vi "test variant to json cluster.vi"(8 "error in (no error)":errorcluster) -> (0 "error out":errorcluster)   [LabVIEW 2019, in "labview_json_tests.lvlib"]
uses:
  labview_json_tests.lvlib
  lib/labview_json.lvlib
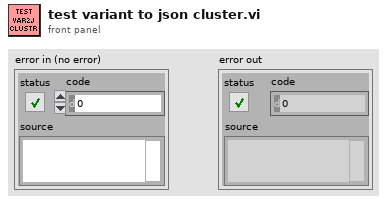
[diagram p1: front panel]
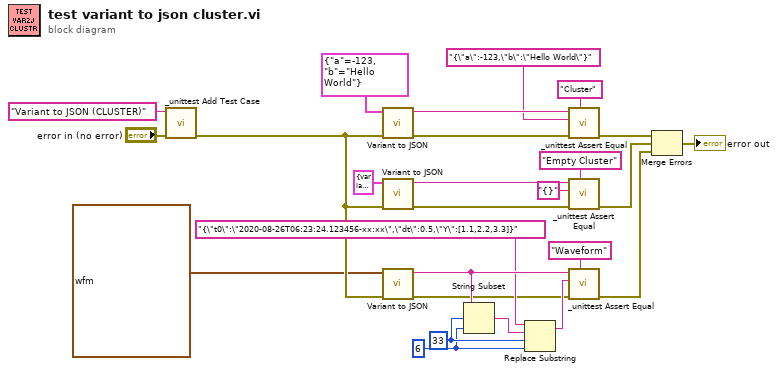
[diagram p0: block diagram]
diagram:
  w5 = 6 ("length (len. of substring)")
  w6 = 33 ("offset (0)")
  n1 = call "_unittest Add Test Case.vi"("error in (no error)"="error in (no error)", "Test Case"="Variant to JSON (CLUSTER)") -> ("error out"=w9:errorcluster)  [unwired: 9 in]
  n2 = call "Variant to JSON.vi"("error in (no error)"=w9, "Variant in"=cluster{"a":i32, "b":string} {"a"=-123, "b"="Hello World"} ("Cluster")) -> ("error out"=w21:errorcluster, "JSON"=w20:string)  [unwired: 8 in]
  n3 = call "Variant to JSON.vi"("error in (no error)"=w9, "Variant in"=cluster{variant} {variant} ("Cluster")) -> ("error out"=w14:errorcluster, "JSON"=w15:string)  [unwired: 8 in]
  n4 = call "Variant to JSON.vi"("error in (no error)"=w9, "Variant in"=waveform(dbl) {"t0"=timestamp(3681289404.123456 s since 1904-01-01), "dt"=0.5, "Y"=[1.1, 2.2, 3.3]} ("Waveform")) -> ("error out"=w1:errorcluster, "JSON"=w7:string)  [unwired: 8 in]
  n5 = String Subset(string=w7, offset (0)=w6, length (rest)=w5) -> (substring=w2:string)
  n6 = Replace Substring(2:w5, 3:w6, 4:w2, 5:"{\"t0\":\"2020-08-26T06:23:24.123456-xx:xx\",\"dt\":0.5,\"Y\":[1.1,2.2,3.3]}") -> (1:w3:string)  [unwired: 1 out]
  n7 = call "_unittest Assert Equal.vi"("Message"="Cluster", "error in (no error)"=w21, "Expected Value"="{\"a\":-123,\"b\":\"Hello World\"}", "Actual Value"=w20) -> ("error out"=w24:errorcluster)  [unwired: 7 in]
  n8 = call "_unittest Assert Equal.vi"("Message"="Empty Cluster", "error in (no error)"=w14, "Expected Value"="{}", "Actual Value"=w15) -> ("error out"=w12:errorcluster)  [unwired: 7 in]
  n9 = call "_unittest Assert Equal.vi"("Message"="Waveform", "error in (no error)"=w1, "Expected Value"=w3, "Actual Value"=w7) -> ("error out"=w10:errorcluster)  [unwired: 7 in]
  n10 = Merge Errors(w24, w12, w10) -> (→"error out":errorcluster)
